vi "Initialize.vi"(5 "components directory (default)":path, 7 "framework options":T1={"FIFO Options"={"Infinite Timeouts"=FALSE}, "Thread Options"={"Show FP On Call"=FALSE, "Close FP After Call"=FALSE, "Allow Debugging"=FALSE}, "Plugin Options"={"Default Components"=FALSE}, "Performance Options"={"Measure Period"=FALSE, "Measure Rx/Tx Duration"=FALSE}, "Data Server Options"={"Enable Data Server"=FALSE, "Period"=100}} {"Data Server Options"."Period" format="%d ms"}, 8 "error in (no error)":errorcluster, 10 "Framework Configuration":refnum<class "Framework Configuration.lvclass">, 11 "Framework in":refnum<class "Framework.lvclass">) -> (0 "error out":errorcluster, 3 "Framework out":refnum<class "Framework.lvclass">)   [LabVIEW 2020, in "DSF Core.lvlib" / "Framework.lvclass"]
uses:
  Framework.lvclass
  Thread/Logging/Logging Thread.lvclass
  Framework States.ctl
  C:/Users/nitest/Desktop/Git/niveristand-data-sharing-framework-custom-device/Source/Core/Classes/Thread/Thread.lvclass
  C:/Users/nitest/Desktop/Git/niveristand-data-sharing-framework-custom-device/Source/Core/Classes/Thread/Logging/Logging Thread.lvclass
  Thread/Dispatcher/Dispatcher Thread.lvclass
  C:/Users/nitest/Desktop/Git/niveristand-data-sharing-framework-custom-device/Source/Core/Classes/Thread/Dispatcher/Dispatcher Thread.lvclass
  Thread/Data Server/Data Server Thread.lvclass
  C:/Users/nitest/Desktop/Git/niveristand-data-sharing-framework-custom-device/Source/Core/Classes/Thread/Data Server/Data Server Thread.lvclass
  Thread/Plugin/Plugin Thread.lvclass
  C:/Users/nitest/Desktop/Git/niveristand-data-sharing-framework-custom-device/Source/Core/Classes/Thread/Plugin/Plugin Thread.lvclass
  Thread/Thread.lvclass
  Typedefs/DSF FIFO Options.ctl
  Thread/Thread Options.ctl
  Framework Options.ctl
  Typedefs/DSF Plugin Options.ctl
  Typedefs/DSF Performance Options.ctl
  DSF Core.lvlib
  Data Server Options.ctl
  Configuration/Core/Framework/Framework Configuration.lvclass
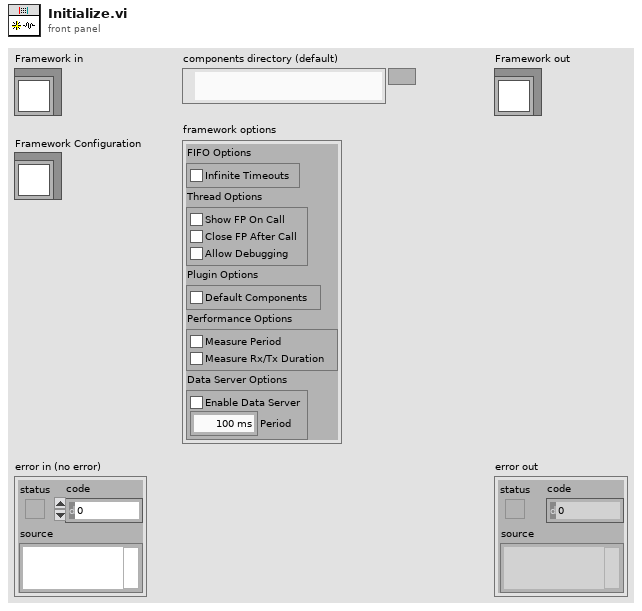
[diagram p1: front panel]
types:
  T1 = typedef "DSF Core.lvlib/Framework.lvclass/Framework Options.ctl" = cluster{"FIFO Options":T2, "Thread Options":T3, "Plugin Options":T4, "Performance Options":T5, "Data Server Options":T6}
  T2 = typedef "DSF Core.lvlib/Framework.lvclass/DSF FIFO Options.ctl" = cluster{"Infinite Timeouts":bool}
  T3 = typedef "DSF Core.lvlib/Thread.lvclass/Thread Options.ctl" = cluster{"Show FP On Call":bool, "Close FP After Call":bool, "Allow Debugging":bool}
  T4 = typedef "DSF Core.lvlib/Framework.lvclass/DSF Plugin Options.ctl" = cluster{"Default Components":bool}
  T5 = typedef "DSF Core.lvlib/DSF Performance Options.ctl" = cluster{"Measure Period":bool, "Measure Rx/Tx Duration":bool}
  T6 = typedef "DSF Core.lvlib/Framework.lvclass/Data Server Options.ctl" = cluster{"Enable Data Server":bool, "Period":u32}
  T7 = typedef "DSF Core.lvlib/Framework.lvclass/Framework States.ctl" = enum8{"Uninitialized", "Initialized", "Start", "Rx", "Tx", "Shutdown"}
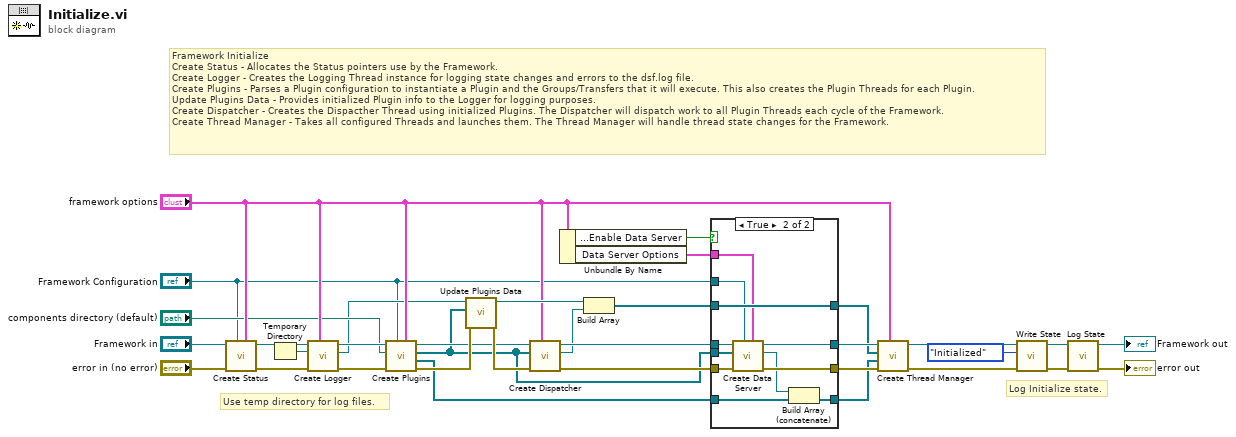
[diagram p0: block diagram]
diagram:
  # "Log Initialize state."
  # "Framework Initialize\nCreate Status - Allocates the Status pointers use by the Framework.\nCreate Logger - Creates the Logging Thread instance for logging state changes and errors to the dsf.log file.\nCreate Plugins - Parses a Plugin configuration to instantiate a Plugin and the Groups/Transfers that it will execute. This also creates the Plugin Threads for each Plugin.\nUpdate Plugins Data - Provides initialized Plugin info to the Logger for logging purposes.\nCreate Dispatcher - Creates the Dispacther Thread using initialized Plugins. The Dispatcher will dispatch work to all Plugin Threads each cycle of the Framework.\nCreate Thread Manager - Takes all configured Threads and launches them. The Thread Manager will handle thread state changes for the Framework."
  # "Use temp directory for log files."
  n1 = call "Create Status.vi"("framework options"="framework options", "Framework Configuration"="Framework Configuration", "error in (no error)"="error in (no error)", "Framework in"="Framework in") -> ("error out"=w29:errorcluster, "Framework out"=w30:refnum<class "Framework.lvclass">)  [unwired: 6 in]
  n2 = Temporary Directory() -> (w26:path)
  n3 = call "Create Logger.vi"("framework options"="framework options", "error in (no error)"=w29, "log file directory"=w26, "Framework in"=w30) -> ("error out"=w27:errorcluster, "Logging Thread"=w3:refnum<class "Logging Thread.lvclass">, "Framework out"=w28:refnum<class "Framework.lvclass">)  [unwired: 4 in, 1 out]
  n4 = call "Create Plugins.vi"("framework options"="framework options", "Framework Configuration"="Framework Configuration", "error in (no error)"=w27, "components directory"="components directory (default)", "Framework in"=w28) -> ("error out"=w33:errorcluster, "Plugin Threads"=w6:refnum<class "Plugin Thread.lvclass">[], "Plugins"=w17:refnum<class "Plugin.lvclass">[], "Framework out"=w32:refnum<class "Framework.lvclass">)  [unwired: 3 in]
  n5 = call "Update Plugins Data.vi"("error in (no error)"=w33, "Plugins"=w17, "Logging Thread in"=w3) -> ("error out"=w34:errorcluster, "Logging Thread out"=w12:refnum<class "Logging Thread.lvclass">)  [unwired: 7 in]
  n6 = call "Create Dispatcher.vi"("framework options"="framework options", "error in (no error)"=w34, "Plugins"=w17, "Framework in"=w32) -> ("error out"=w18:errorcluster, "Dispatcher Thread"=w11:refnum<class "Dispatcher Thread.lvclass">, "Framework out"=w16:refnum<class "Framework.lvclass">)  [unwired: 5 in]
  n7 = Unbundle By Name("framework options") -> ("Data Server Options.Enable Data Server"=w7:bool, "Data Server Options"=w8:T6)
  n8 = Build Array(w12, w11) -> (w10:refnum<class "Thread.lvclass">[])
  n9 = case shown="True" w7 {
    tunnel: w18 -> [w36 w49]
    tunnel: w17 -> [_ w48]
    tunnel: w16 -> [w37 w47]
    tunnel: [w37 w46] -> w15
    tunnel: [w38 w44] -> w14
    tunnel: [w36 w45] -> w13
    tunnel: w10 -> [w38 w44]
    tunnel: w8 -> [_ w40]
    tunnel: w6 -> [w35 w41]
    tunnel: [w35 w43] -> w5
    tunnel: "Framework Configuration" -> [_ w39]
    frame False {
    }
    frame True {
      n10 = call "Create Data Server.vi"("data server options"=w40, "Framework Configuration"=w39, "error in (no error)"=w49, "Plugins"=w48, "Framework in"=w47) -> ("error out"=w45:errorcluster, "Data Server Thread"=w42:refnum<class "Data Server Thread.lvclass">, "Framework out"=w46:refnum<class "Framework.lvclass">)  [unwired: 4 in]
      n11 = Build Array (concatenate)(w42, w41) -> (w43:refnum<class "Thread.lvclass">[])
    }
  }
  n12 = call "Create Thread Manager.vi"("framework options"="framework options", "error in (no error)"=w13, "Public Threads"=w5, "Private Threads"=w14, "Framework in"=w15) -> ("error out"=w24:errorcluster, "Framework out"=w25:refnum<class "Framework.lvclass">)  [unwired: 5 in]
  n13 = call "Write State.vi"("error in (no error)"=w24, "state"=Framework_States."Initialized", "Framework in"=w25) -> ("error out"=w21:errorcluster, "Framework out"=w22:refnum<class "Framework.lvclass">)  [unwired: 7 in]
  n14 = call "Log State.vi"("error in (no error)"=w21, "Framework in"=w22) -> ("error out"=→"error out":errorcluster, "Framework out"=→"Framework out":refnum<class "Framework.lvclass">)  [unwired: 8 in]
